vi "TEST - List VI Hierarchy.vi"(8 "error in (no error)":errorcluster) -> (0 "error out":errorcluster, 2 "pass":bool)   [LabVIEW 2009]
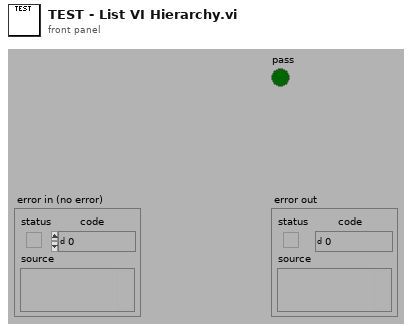
[diagram p1: front panel]
types:
  T1 = cluster{"Standard VIs":string[], "Control Type Definitions":string[], "Global VIs":string[], "Polymorphic VIs":string[]}
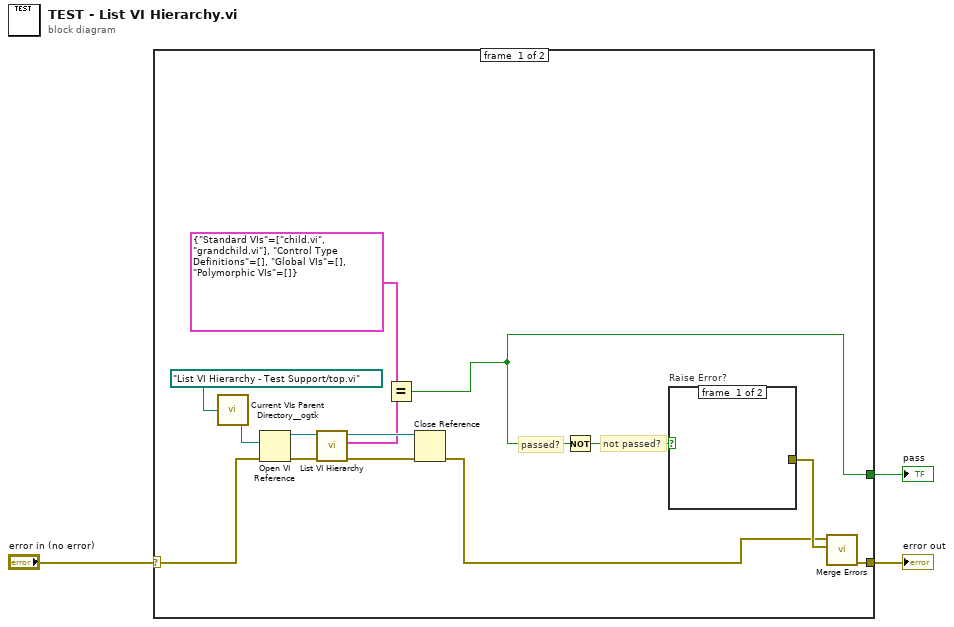
[diagram p0: block diagram]
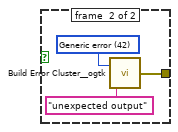
[diagram p2: hidden frame]
diagram:
  n1 = case shown="No Error" "error in (no error)" {
    selector: "error in (no error)" -> [w7 w21]
    tunnel: [w4 _] -> w3
    tunnel: [w17 w21] -> w1
    frame #0 {
      # "not passed?"
      # "passed?"
      n2 = call <userlib>:"Current VIs Parent Directory__ogtk.vi"("Relative path (.)"=path "List VI Hierarchy - Test Support/top.vi") -> ("Parent Directory (+ Relative)"=w11:path)  [unwired: 4 in]
      n3 = Open VI Reference(vi path=w11, error in (no error)=w7) -> (vi reference=w12:refnum<vi>, error out=w13:errorcluster)  [unwired: 4 in]
      n4 = call "List VI Hierarchy.vi"("error in (no error)"=w13, "VI reference"=w12) -> ("error out"=w9:errorcluster, "Hierarchy Lists"=w6:T1, "dup VI reference"=w10:refnum<vi>)  [unwired: 7 in]
      n5 = Equal?(x=T1 {"Standard VIs"=["child.vi", "grandchild.vi"], "Control Type Definitions"=[], "Global VIs"=[], "Polymorphic VIs"=[]} ("Hierarchy Lists"), y=w6) -> (x = y?=w4:bool)
      n6 = Close Reference(reference=w10, error in (no error)=w9) -> (error out=w8:errorcluster)
      n7 = Not(x=w4) -> (.not. x?=w15:bool)
      n8 = case "Raise Error?" shown="True" w15 {
        tunnel: [_ w18] -> w16
        frame #0 {
        }
        frame #1 {
          w19 = 42 items=["No error", "Argument error", "Memory is full", "Out of zone", "End of file", "File already open", "Generic file I/O error", "File not found", "File permission error", "Disk is full", "Duplicate path", "Too many files open", "System feature not enabled", "Resource file not found", "Cannot add resource", "Resource not found", "Image not found", "Image memory error", "Pen does not exist", "Config type invalid", "Config token not found", "Config parse error", "Config memory error", "Bad external code format", "Bad external code offset", "External code not present", "Null window", "Destroy window error", "Null menu", "Print aborted", "Bad print record", "Print driver error", "Windows error during printing", "Memory error during printing", "Print dialog error", "Generic print error", "Invalid device refnum", "Device not found", "Device parameter error", "Device unit error", "Cannot open device", "Device call aborted", "Generic error", "Cancelled by user", "Object ID too low", "Object ID too high", "Object not in heap", "Unknown heap", "Unknown object (invalid DefProc)", "Unknown object (DefProc not in table)", "Message out of range", "Invalid (null) method", "Unknown message", "Manager call not supported", "Bad address", "Network operation in progress", "Network operation timed out", "Connection is busy", "Network attribute not supported", "Network error", "Address in use", "System out of memory", "Connection aborted", "Connection refused", "Not connected", "Already connected", "Connection closed", "Initialization error (interapplication manager)", "Bad occurrence", "Wait on unbound occurrence handler", "Occurrence queue overflow", "Datalog type conflict", "Unused", "Unrecognized type (interapplication manager)", "Memory corrupt", "Failed to make temporary DLL", "Old CIN version", "Drag socket not found", "Failed to load drop-object", "Failed to register OLE object", "Failed to release OLE object", "Format specifier type mismatch", "Unknown format specifier", "Too few format specifiers", "Too many format specifiers", "Scan failed", "Newer CIN version", "Error converting to variant", "Runtime menu error", "Password tampered", "Variant attribute not found", "Incompatible variant data type", "Event data is not available", "Event Store is not present", "Occurrence is not found", "Event Queue is not created", "Event info is not available", "Refnum passed is NULL", "Error retrieving Class GUID", "Error retrieving CoClass GUID", "Error retrieving TypeLib GUID.", "Bad built application magic bytes.", "Specific driver is different from the specific driver associated with the Logical Name.", "There is no session opened to the class driver.", "Max Error", "MAX - Error with config objects", "MAX - Error loading configuration", "MAX - Group not supported"]
          n9 = call <userlib>:"Build Error Cluster__ogtk.vi"("String to Prepend to source (\"\")"="unexpected output" ("String to Prepend to source (\"\")"), "code"=w19) -> ("error out"=w18:errorcluster)
        }
      }
      n10 = call <vilib>:"Merge Errors.vi"("error in 2 (no error)"=w16, "error in 1 (no error)"=w8) -> ("error out"=w17:errorcluster)  [unwired: 5 in]
    }
    frame #1 {
    }
  }
  "pass" <- w3
  "error out" <- w1
